vi "Check Path.vi"(8 "error in (no error)":errorcluster, 10 "appended array":path[](array[path])) -> (0 "error in (no error)":errorcluster, 2 "Library Path":path)   [LabVIEW 2020, in "lvzstd.lvlib"]
uses:
  lvzstd.lvlib
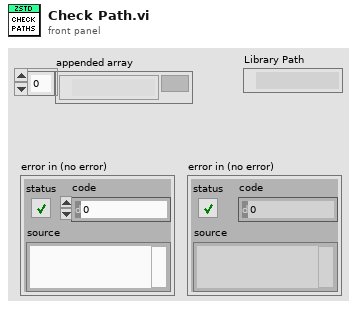
[diagram p1: front panel]
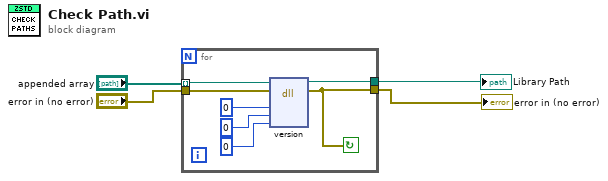
[diagram p0: block diagram]
diagram:
  n1 = for {
    tunnel: "appended array" -> [w8] mode=indexing
    tunnel: [w7] -> w4
    tunnel: [w6] -> w1
    tunnel: "error in (no error)" -> [w5]
    stop <- w7 continue-if-true
    n2 = dll-call lib="?" fn="version"(path in=w8, error in=w5, "major"=0, "minor"=0, "patch"=0) -> (path out=w6:path, error out=w7:errorcluster)  [unwired: 5 in]
  }
  "error in (no error)" <- w4
  "Library Path" <- w1
